vi "Validate Default State.vi"(8 "error in (no error)":errorcluster, 11 "Plugin_UI in":refnum<class "Plugin_UI.lvclass">) -> (0 "error out":errorcluster, 1 "Error message":string, 2 "Conflicts in Default State?":bool, 3 "Plugin_UI out":refnum<class "Plugin_UI.lvclass">)   [LabVIEW 2020, in "Plugin.lvlib" / "Plugin_UI.lvclass"]
doc: "Validate the channel consistency of the default state."
uses:
  Plugin_UI.lvclass
  C:/SVN_LabSys/labsys_lvcode/LabSys_SourceCode/builds/Libraries/LabSys Framework.lvlibp/Configurable Data Node/Configuration Interface/Configuration Interface.lvclass
  builds/Libraries/Shared GUI Library.lvlibp/Shared GUI Library/Channel redundancy check/Type defs/channel check.ctl
  Plugin_UI.lvclass/Plugin_UI.ctl
  Read Output Channels[].vi
  Read Input Channels[].vi
  Channels/Output Channels/Output Channels.lvclass
  C:/SVN_LabSys/labsys_lvcode/LabSys_SourceCode/Plugin Template/Source/Code/Channels/Plugin_Channels.lvclass
  Channels/Input Channels/Input Channels.lvclass
  builds/Libraries/LabSys Framework.lvlibp/Configurable Data Node/Configuration Interface/Read Module Configuration.vi
  builds/Libraries/LabSys Framework.lvlibp/Configurable Data Node/Configuration Interface/Write Module Configuration.vi
  builds/Libraries/LabSys Framework.lvlibp/Configuration Storage/Module Configuration/Module Configuration.lvclass
  builds/Libraries/Shared GUI Library.lvlibp
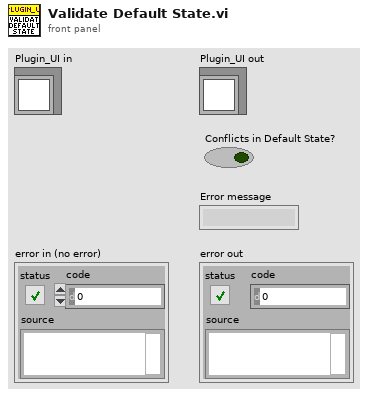
[diagram p1: front panel]
types:
  T1 = typedef "Shared GUI Library.lvlibp/channel check.ctl" = enum16{"All Check", "Charcheck", "InternalNameCheck", "ExternalNameCheck"}
  T2 = typedef "Plugin.lvlib/Plugin_UI.lvclass/UDP Configuration.ctl" = cluster{"Device Port Number":u16, "Device IP":string, "Timeout":i32, "Port Number":u16}
  T3 = typedef "Plugin.lvlib/Plugin_UI.lvclass/Serial Configuration.ctl" = cluster{"VISA":refnum<visa-resource-name>, "Interface Type":T4, "Serial Interface":T5, "Slave Address":u8}
  T4 = typedef "Shared GUI Library.lvlibp/Interface Type.ctl" = u16
  T5 = typedef "Shared GUI Library.lvlibp/Serial Interafce.ctl" = cluster{"Baud Rate":u32, "Data Bits ":u16, "Parity":enum16{"None", "Odd", "Even"}, "Stop Bits":u16}
  T6 = typedef "Plugin.lvlib/Plugin_UI.lvclass/Output Channel Config.ctl" = cluster{"Enable Output":bool, "Channel Name":string, "Value":dbl, "Unit":string}
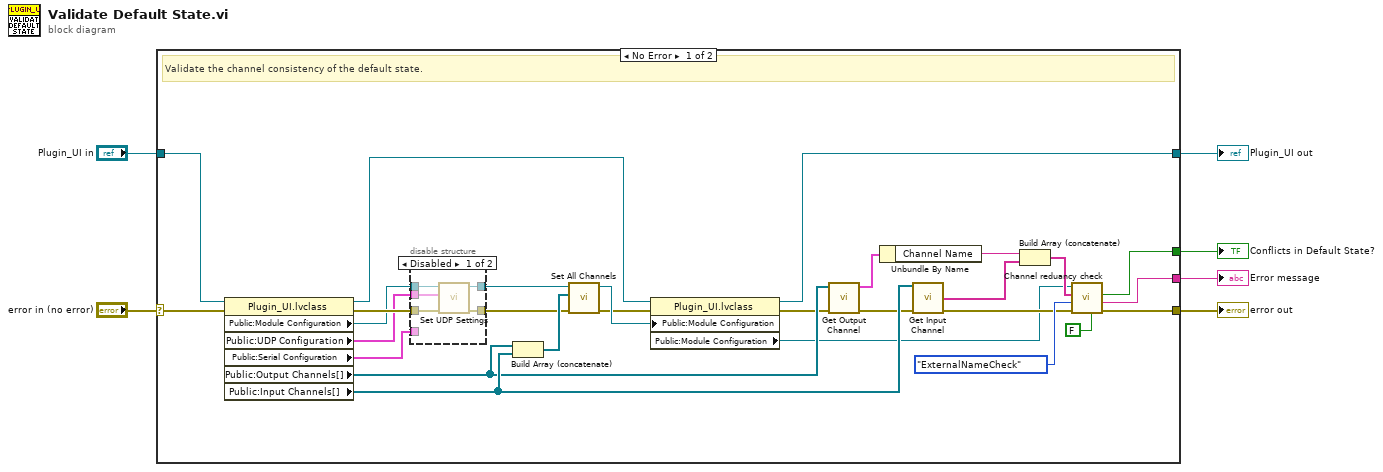
[diagram p0: block diagram]
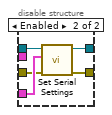
[diagram p2: hidden frame]
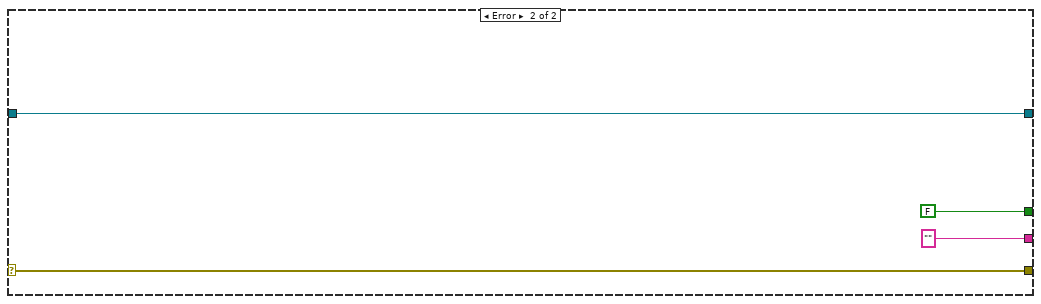
[diagram p3: hidden frame]
diagram:
  n1 = case shown="No Error" "error in (no error)" {
    selector: "error in (no error)" -> [w10 w48]
    tunnel: [w34 "" ("Error message")] -> w6
    tunnel: [w33 FALSE ("Channel Configuration Found(F)")] -> w5
    tunnel: [w32 w48] -> w4
    tunnel: [w17 w45] -> w3
    tunnel: "Plugin_UI in" -> [w16 w45]
    frame No Error {
      # "Validate the channel consistency of the default state."
      n2 = property class="Plugin_UI.lvclass"(reference=w16, error in=w10) -> (reference out=w15:refnum<class "Plugin_UI.lvclass">, error out=w14:errorcluster, "Public:Module Configuration"=w12:refnum<class "Module Configuration.lvclass">, "Public:UDP Configuration"=w13:T2, "Public:Serial Configuration"=w9:T3, "Public:Output Channels[]"=w25:refnum<class "Output Channels.lvclass">[], "Public:Input Channels[]"=w26:refnum<class "Input Channels.lvclass">[])
      n3 = disable-structure shown="Disabled" {
        disable-tunnel: w14 -> [w39 w40]
        disable-tunnel: w13 -> [w38 _]
        disable-tunnel: w12 -> [w37 w42]
        disable-tunnel: [w36 w44] -> w11
        disable-tunnel: [w35 w43] -> w8
        disable-tunnel: w9 -> [_ w41]
        frame Disabled {
          n4 = call "Set UDP Settings.vi"("error in (no error)"=w39, "Hardware Configuration"=w38, "Module Configuration"=w37) -> ("error out"=w36:errorcluster, "Module Configuration out"=w35:refnum<class "Module Configuration.lvclass">)  [unwired: 7 in]
        }
        frame Enabled {
          n5 = call "Set Serial Settings.vi"("error IO"=w40, "Serial Configuration"=w41, "Module Configuration"=w42) -> ("error IO out"=w44:errorcluster, "Module Configuration out"=w43:refnum<class "Module Configuration.lvclass">)  [unwired: 7 in]
        }
      }
      n6 = Build Array (concatenate)(w25, w26) -> (w18:refnum<class "Plugin_Channels.lvclass">[])
      n7 = call "Set All Channels.vi"("error in"=w11, "Channels[]"=w18, "Module Configuration in"=w8) -> ("error out"=w19:errorcluster, "Module Configuration out"=w20:refnum<class "Module Configuration.lvclass">)  [unwired: 7 in]
      n8 = property class="Plugin_UI.lvclass"(reference=w15, error in=w19, "Public:Module Configuration"=w20) -> (reference out=w17:refnum<class "Plugin_UI.lvclass">, error out=w22:errorcluster, "Public:Module Configuration"=w21:refnum<class "Module Configuration.lvclass">)
      n9 = call "Get Output Channel.vi"("error in (no error)"=w22, "Output Channels[]"=w25) -> ("error out"=w23:errorcluster, "Output Channel Details"=w27:T6)  [unwired: 8 in]
      n10 = Unbundle By Name(w27) -> ("Channel Name"=w28:string)
      n11 = call "Get Input Channel.vi"("Input Channels[]"=w26, "error in (no error)"=w23) -> ("Active Channels[]"=w7:string[], "error out"=w24:errorcluster)  [unwired: 7 in, 5 out]
      n12 = Build Array (concatenate)(w28, w7) -> (w29:string[])
      n13 = call "Channel reduancy check.vi"("Show Pop up"=FALSE, "error in"=w24, "Check Function"=channel_check."ExternalNameCheck", "New Channel Name[]"=w29, "Module configuration in"=w21) -> ("error out"=w32:errorcluster, "Error message"=w34:string, "Channel Configuration Found(F)"=w33:bool)  [unwired: 3 in, 1 out]
    }
    frame Error {
    }
  }
  "Error message" <- w6
  "Conflicts in Default State?" <- w5
  "error out" <- w4
  "Plugin_UI out" <- w3
